vi "Two Ball Atonomous.vi"(0 "Intake Roller Speed":dbl(knob) scale=-1.0..1.0, 1 "Move Forward speed":dbl(knob) scale=-1.0..1.0, 2 "Rolling Speed":dbl(knob) scale=-1.0..1.0, 3 "Gyro Margin":dbl, 4 "Move Forward distance":dbl, 5 "Right Angle":dbl, 6 "Left Angle":dbl) -> ()   [LabVIEW 2013]
panel:
  # "Intake motor value for rolling a ball behind us"
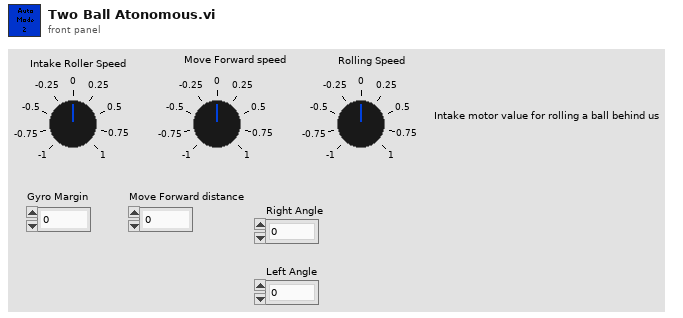
[diagram p1: front panel]
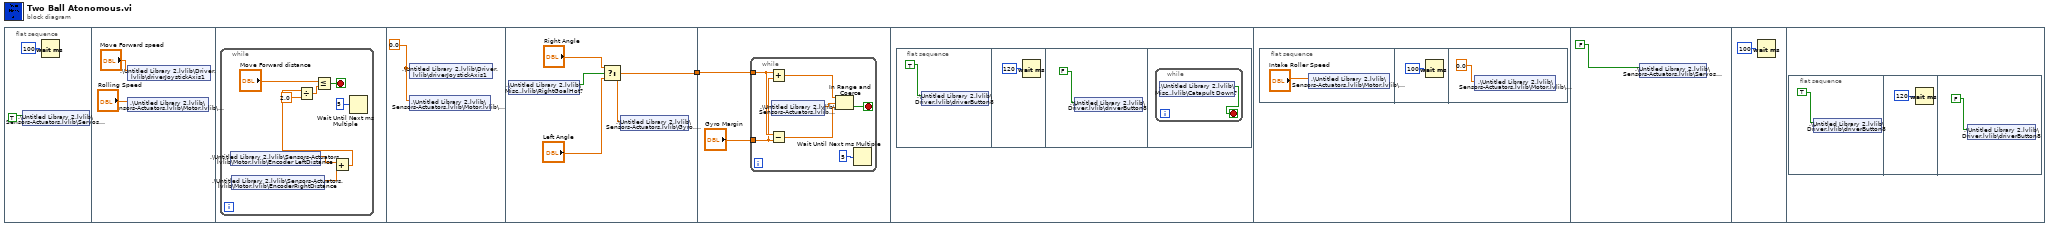
[diagram p0: block diagram]
diagram:
  n1 = flat-sequence {
    tunnel: [w15] -> w1
    tunnel: w1 -> [w20]
    frame #0 {
      n2 = shared-variable ".\\Untitled Library 2.lvlib\\Sensors-Actuators.lvlib\\Servos.lvlib\\Intake Down?"(TRUE ("Intake Arm Position")) -> ()  [unwired: 1 in, 1 out]
      n3 = Wait (ms)(milliseconds to wait=u32 100) -> ()  [unwired: 1 out]
    }
    frame #1 {
      n4 = shared-variable ".\\Untitled Library 2.lvlib\\Driver.lvlib\\driverJoystickAxis1"("Move Forward speed") -> ()  [unwired: 1 in, 1 out]
      n5 = shared-variable ".\\Untitled Library 2.lvlib\\Sensors-Actuators.lvlib\\Motor.lvlib\\IntakeMotorValue"("Rolling Speed") -> ()  [unwired: 1 in, 1 out]
    }
    frame #2 {
      n6 = while {
        stop <- w12 stop-if-true
        n7 = shared-variable ".\\Untitled Library 2.lvlib\\Sensors-Actuators.lvlib\\Motor.lvlib\\Encoder LeftDistance"() -> (w10:dbl)  [unwired: 1 in, 1 out]
        n8 = shared-variable ".\\Untitled Library 2.lvlib\\Sensors-Actuators.lvlib\\Motor.lvlib\\EncoderRightDistance"() -> (w9:dbl)  [unwired: 1 in, 1 out]
        n9 = Add(x=w10, y=w9) -> (x+y=w7:dbl)
        n10 = Divide(x=w7, y=2.0) -> (x/y=w8:dbl)
        n11 = Less Or Equal?(x="Move Forward distance", y=w8) -> (x <= y?=w12:bool)
        n12 = Wait Until Next ms Multiple(millisecond multiple=u32 5) -> ()  [unwired: 1 out]
      }
    }
    frame #3 {
      w14 = 0.0 ("Speed")
      n13 = shared-variable ".\\Untitled Library 2.lvlib\\Driver.lvlib\\driverJoystickAxis1"(w14) -> ()  [unwired: 1 in, 1 out]
      n14 = shared-variable ".\\Untitled Library 2.lvlib\\Sensors-Actuators.lvlib\\Motor.lvlib\\IntakeMotorValue"(w14) -> ()  [unwired: 1 in, 1 out]
    }
    frame #4 {
      n15 = shared-variable ".\\Untitled Library 2.lvlib\\Misc..lvlib\\RightGoalHot?"() -> (w16:bool)  [unwired: 1 in, 1 out]
      n16 = Select(t="Right Angle", s=w16, f="Left Angle") -> (s? t:f=w15:dbl)
      n17 = shared-variable ".\\Untitled Library 2.lvlib\\Sensors-Actuators.lvlib\\Gyro.lvlib\\Desired Angle"(w15) -> ()  [unwired: 1 in, 1 out]
    }
    frame #5 {
      n18 = while {
        tunnel: w20 -> [w27]
        tunnel: "Gyro Margin" -> [w26]
        stop <- w25 stop-if-true
        n19 = Add(x=w27, y=w26) -> (x+y=w24:dbl)
        n20 = Subtract(x=w27, y=w26) -> (x-y=w23:dbl)
        n21 = shared-variable ".\\Untitled Library 2.lvlib\\Sensors-Actuators.lvlib\\Gyro.lvlib\\yawGyro"() -> (w21:dbl)  [unwired: 1 in, 1 out]
        n22 = In Range and Coerce(upper limit=w24, x=w21, lower limit=w23) -> (In Range?=w25:bool)  [unwired: 1 out]
        n23 = Wait Until Next ms Multiple(millisecond multiple=u32 5) -> ()  [unwired: 1 out]
      }
    }
    frame #6 {
      n24 = flat-sequence {
        frame #0 {
          n25 = shared-variable ".\\Untitled Library 2.lvlib\\Driver.lvlib\\driverButton8"(TRUE) -> ()  [unwired: 1 in, 1 out]
        }
        frame #1 {
          n26 = Wait (ms)(milliseconds to wait=u32 120) -> ()  [unwired: 1 out]
        }
        frame #2 {
          n27 = shared-variable ".\\Untitled Library 2.lvlib\\Driver.lvlib\\driverButton8"(FALSE) -> ()  [unwired: 1 in, 1 out]
        }
        frame #3 {
          n28 = while {
            stop <- w31 stop-if-true
            n29 = shared-variable ".\\Untitled Library 2.lvlib\\Misc..lvlib\\Catapult Down?"() -> (w31:bool)  [unwired: 1 in, 1 out]
          }
        }
      }
    }
    frame #7 {
      n30 = flat-sequence {
        frame #0 {
          n31 = shared-variable ".\\Untitled Library 2.lvlib\\Sensors-Actuators.lvlib\\Motor.lvlib\\IntakeMotorValue"("Intake Roller Speed") -> ()  [unwired: 1 in, 1 out]
        }
        frame #1 {
          n32 = Wait (ms)(milliseconds to wait=u32 100) -> ()  [unwired: 1 out]
        }
        frame #2 {
          n33 = shared-variable ".\\Untitled Library 2.lvlib\\Sensors-Actuators.lvlib\\Motor.lvlib\\IntakeMotorValue"(0.0 ("Intake Motor")) -> ()  [unwired: 1 in, 1 out]
        }
      }
    }
    frame #8 {
      n34 = shared-variable ".\\Untitled Library 2.lvlib\\Sensors-Actuators.lvlib\\Servos.lvlib\\Intake Down?"(FALSE ("Intake Arm Position\nLit Up / Not Down")) -> ()  [unwired: 1 in, 1 out]
    }
    frame #9 {
      n35 = Wait (ms)(milliseconds to wait=u32 100) -> ()  [unwired: 1 out]
    }
    frame #10 {
      n36 = flat-sequence {
        frame #0 {
          n37 = shared-variable ".\\Untitled Library 2.lvlib\\Driver.lvlib\\driverButton8"(TRUE) -> ()  [unwired: 1 in, 1 out]
        }
        frame #1 {
          n38 = Wait (ms)(milliseconds to wait=u32 120) -> ()  [unwired: 1 out]
        }
        frame #2 {
          n39 = shared-variable ".\\Untitled Library 2.lvlib\\Driver.lvlib\\driverButton8"(FALSE) -> ()  [unwired: 1 in, 1 out]
        }
      }
    }
  }
